vi "Read Joystick.vi"(9 "Joystick Input":T1, 11 "Joystick String":string="My Joystick RefNum") -> (1 "Joystick Output":T1)   [LabVIEW 2011]
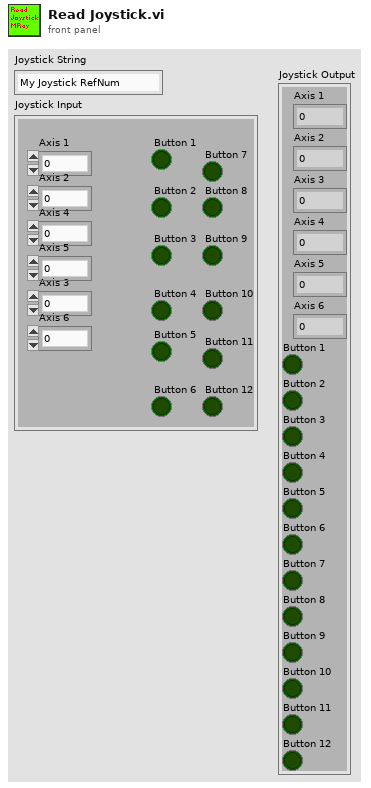
[diagram p1: front panel]
types:
  T1 = cluster{"Axis 1":dbl, "Axis 2":dbl, "Axis 3":dbl, "Axis 4":dbl, "Axis 5":dbl, "Axis 6":dbl, "Button 1":bool, "Button 2":bool, "Button 3":bool, "Button 4":bool, "Button 5":bool, "Button 6":bool, "Button 7":bool, "Button 8":bool, "Button 9":bool, "Button 10":bool, "Button 11":bool, "Button 12":bool}
  T2 = typedef "WPI_JoystickDevRef.ctl" = cluster{"Device":T3}
  T3 = typedef "WPI_JoystickDeviceEnum.ctl" = enum16{"USB 1", "USB 2", "USB 3", "USB 4", "Kinect 1", "Kinect 2"}
  T4 = typedef "WPI_JoystickButtonState.ctl" = cluster{"Button 1":bool, "Button 2":bool, "Button 3":bool, "Button 4":bool, "Button 5":bool, "Button 6":bool, "Button 7":bool, "Button 8":bool, "Button 9":bool, "Button 10":bool, "Button 11":bool, "Button 12":bool}
  T5 = cluster{"axis 1 (x)":dbl, "axis 2 (y)":dbl, "axis 3 (throttle)":dbl, "axis 4":dbl, "axis 5":dbl, "axis 6":dbl}
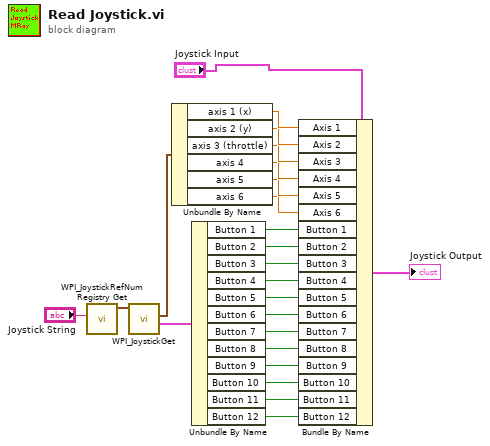
[diagram p0: block diagram]
diagram:
  n1 = call <vilib>:"WPI_JoystickRefNum Registry Get.vi"("refnum name"="Joystick String") -> ("JoystickDevRef"=w23:T2)  [unwired: 9 in, 1 out]
  n2 = call <vilib>:"WPI_JoystickGet.vi"("JoystickDevRef"=w23) -> ("Buttons"=w21:T4, "Axes"=w22:T5)  [unwired: 4 in, 1 out]
  n3 = Unbundle By Name(w22) -> ("axis 1 (x)"=w20:dbl, "axis 2 (y)"=w19:dbl, "axis 3 (throttle)"=w18:dbl, "axis 4"=w17:dbl, "axis 5"=w16:dbl, "axis 6"=w15:dbl)
  n4 = Unbundle By Name(w21) -> ("Button 1"=w14:bool, "Button 2"=w13:bool, "Button 3"=w12:bool, "Button 4"=w11:bool, "Button 5"=w10:bool, "Button 6"=w9:bool, "Button 7"=w8:bool, "Button 8"=w7:bool, "Button 9"=w6:bool, "Button 10"=w5:bool, "Button 11"=w4:bool, "Button 12"=w3:bool)
  n5 = Bundle By Name(cluster="Joystick Input", "Axis 1"=w20, "Axis 2"=w19, "Axis 3"=w18, "Axis 4"=w17, "Axis 5"=w16, "Axis 6"=w15, "Button 1"=w14, "Button 2"=w13, "Button 3"=w12, "Button 4"=w11, "Button 5"=w10, "Button 6"=w9, "Button 7"=w8, "Button 8"=w7, "Button 9"=w6, "Button 10"=w5, "Button 11"=w4, "Button 12"=w3) -> (→"Joystick Output":T1)
